vi "Read Serial Config.vi"(8 "error in (no error)":errorcluster, 11 "Rabbit BL2610 in":refnum<class "MB PLC Client.lvclass">) -> (0 "error out":errorcluster, 2 "Serial Config":T1={"COM Port"="", "Slave ID"=255, "baud rate (bps)"=19200, "Mode"=enum."RTU", "Parity"=0, "Flow Control"=0, "Timeout"=10000, "Retries"=255, "Stop Bits"=10} {"Stop Bits" items=["1.0"=10, "1.5"=15, "2.0"=20]; "Flow Control" items=["None", "XON/XOFF", "RTS/CTS", "XON/XOFF & RTS/CTS", "DTR/DSR", "XON/XOFF & DTR/DSR"]; "Parity" items=["None", "Odd", "Even", "Mark", "Space"]}, 3 "Rabbit BL2610 out":refnum<class "MB PLC Client.lvclass">)   [LabVIEW 2018, in "MB PLC Client.lvlib" / "MB PLC Client.lvclass"]
uses:
  MB PLC Client.lvclass
  Types/Serial Config_Cluster.ctl
  MB PLC Client.lvclass/MB PLC Client.ctl
  MB PLC Client.lvlib
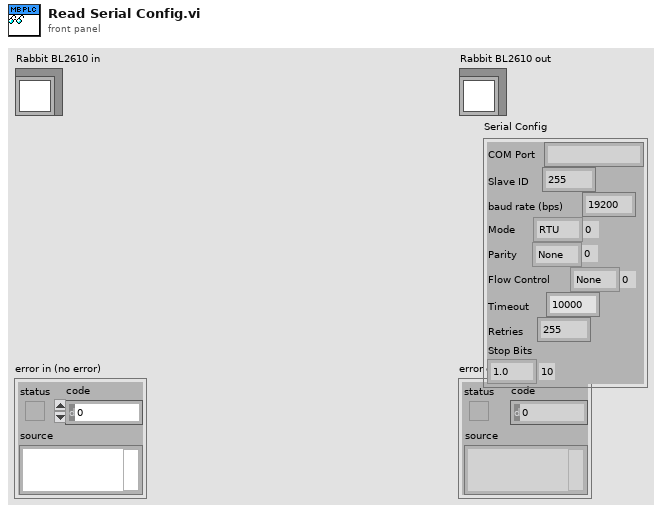
[diagram p1: front panel]
types:
  T1 = typedef "MB PLC Client.lvlib/Serial Config_Cluster.ctl" = cluster{"COM Port":string, "Slave ID":u8, "baud rate (bps)":u32, "Mode":enum16{"RTU", "ASCII"}, "Parity":u16, "Flow Control":u16, "Timeout":u32, "Retries":u8, "Stop Bits":u16}
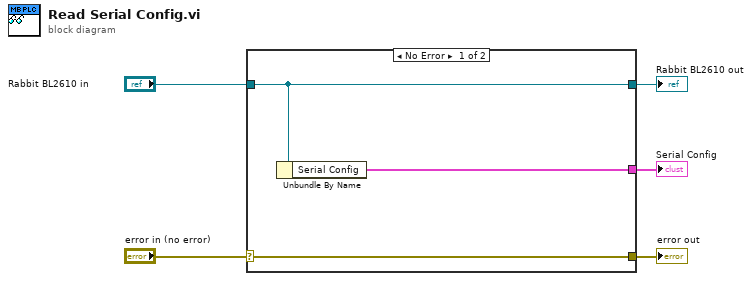
[diagram p0: block diagram]
diagram:
  n1 = case shown="No Error" "error in (no error)" {
    selector: "error in (no error)" -> [w8 w9]
    tunnel: [w8 w9] -> w4
    tunnel: [w7 w10] -> w2
    tunnel: "Rabbit BL2610 in" -> [w7 w10]
    tunnel: [w6 _] -> w1
    frame No Error {
      n2 = Unbundle By Name(w7) -> ("Serial Config"=w6:T1)
    }
    frame Error {
    }
  }
  "error out" <- w4
  "Rabbit BL2610 out" <- w2
  "Serial Config" <- w1
